vi "Find_Full_Equal_Points-1.vi"(4 "error IN":errorcluster, 5 "[IN] Activate Search???":bool, 7 "[IN] Clusters for Re\nconstructed Tracks":T1) -> (0 "error OUT":errorcluster, 3 "[OUT] Clusters for Re\nconstructed Tracks":T1)   [LabVIEW 2017]
panel:
  out "# of Track":i32
  out "Index in Track":i32
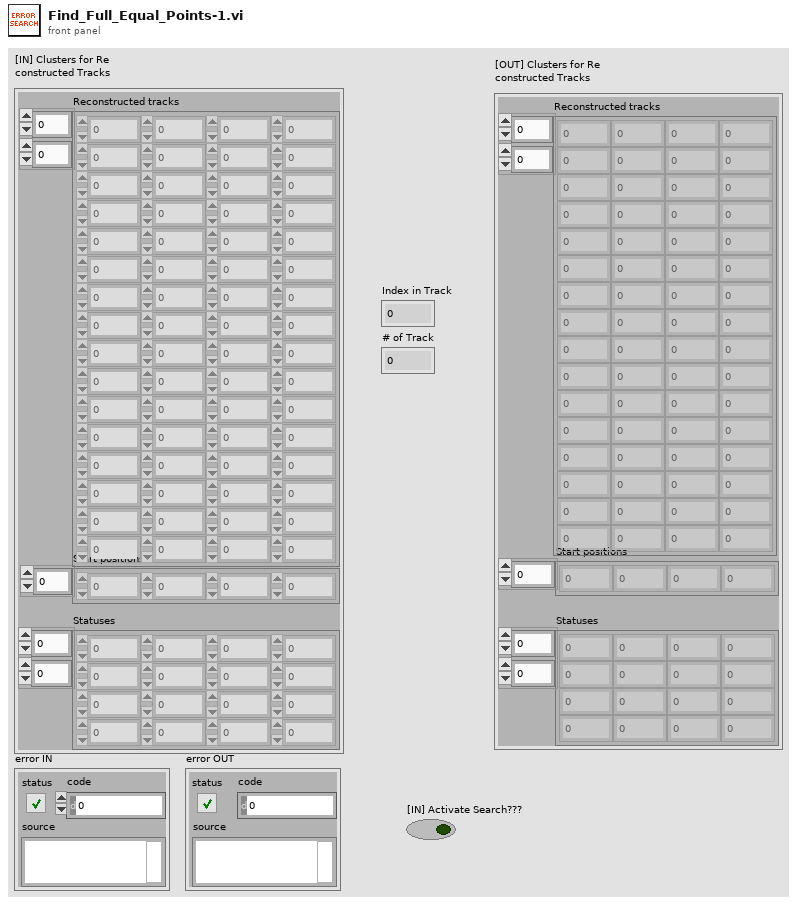
[diagram p1: front panel]
types:
  T1 = cluster{"Reconstructed tracks":dbl[][], "Start positions":i32[], "Statuses":i16[][]}
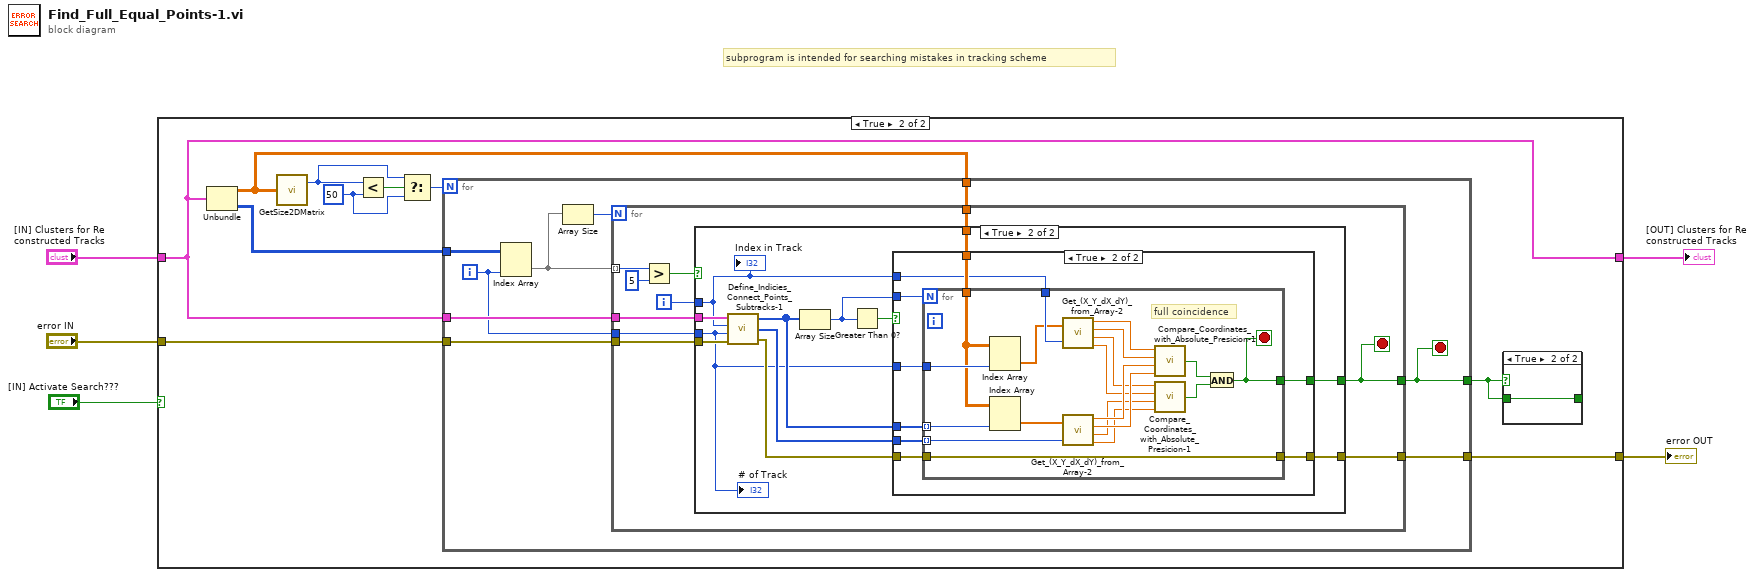
[diagram p0: block diagram]
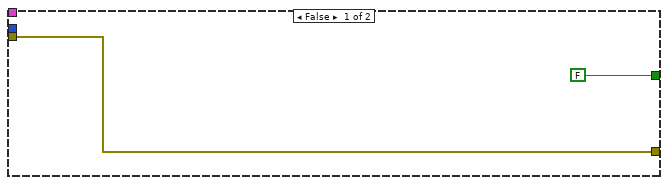
[diagram p4: hidden frame]
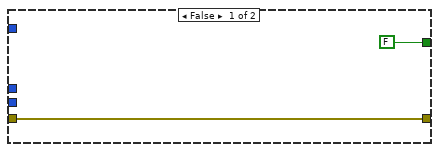
[diagram p5: hidden frame]
diagram:
  # "subprogram is intended for searching mistakes in tracking scheme"
  n1 = case shown="True" "[IN] Activate Search???" {
    tunnel: "[IN] Clusters for Re\nconstructed Tracks" -> [w6 w8]
    tunnel: "error IN" -> [w7 w12]
    tunnel: [w7 w10] -> w2
    tunnel: [w6 w8] -> w1
    frame False {
    }
    frame True {
      w15 = 50 ("y")
      n2 = Unbundle(w8) -> ("Reconstructed tracks"=w11:dbl[][], "Statuses"=w13:i16[][])  [unwired: 1 out]
      n3 = call "GetSize2DMatrix.vi"("Array IN (2D)"=w11) -> ("# Cols"=w16:i32)  [unwired: 1 out]
      n4 = Less?(x=w16, y=w15) -> (x < y?=w17:bool)
      n5 = Select(t=w16, s=w17, f=w15) -> (s? t:f=w14:i32)
      n6 = for {
        N: w14 -> [_]
        tunnel: w13 -> [w28]
        tunnel: w8 -> [w25]
        tunnel: w12 -> [w24]
        tunnel: w11 -> [w22]
        tunnel: [w21] -> w9
        tunnel: [w20] -> w10
        i -> [w23]
        stop <- w21 stop-if-true
        n7 = Index Array(array=w28, index (col)=w23) -> (element=w26:i16[])  [unwired: 1 in]
        n8 = Array Size(array=w26) -> (size(s)=w27:i32)
        n9 = for {
          N: w27 -> [_]
          tunnel: w26 -> [w34] mode=indexing
          tunnel: w25 -> [w36]
          tunnel: w24 -> [w35]
          tunnel: w23 -> [w32]
          tunnel: w22 -> [w31]
          tunnel: [w30] -> w21
          tunnel: [w29] -> w20
          i -> [w33]
          stop <- w30 stop-if-true
          n10 = Greater?(x=w34, y=i16 5) -> (0:w37:bool)
          n11 = case shown="True" w37 {
            tunnel: w36 -> [_ w52]
            tunnel: w35 -> [w39 w51]
            tunnel: w33 -> [_ w43]
            tunnel: w32 -> [_ w44]
            tunnel: w31 -> [_ w45]
            tunnel: [FALSE w42] -> w30
            tunnel: [w39 w41] -> w29
            frame False {
            }
            frame True {
              n12 = call "Define_Indicies_Connect_Points_Subtracks-1.vi"("error IN"=w51, "[IN] Index of track with\n(problem displacement)"=w44, "[IN] Index of problem\ndisplacement inside track"=w43, "[IN] Track group"=w52) -> ("error OUT"=w46:errorcluster, "[OUT] Index of \nconnected dots\ninside the track"=w47:i32[], "[OUT] Index of connected\ntracks with problem dot"=w48:i32[])
              n13 = Array Size(array=w48) -> (size(s)=w50:i32)
              n14 = Greater Than 0?(x=w50) -> (x > 0?=w49:bool)
              n15 = case shown="True" w49 {
                tunnel: w50 -> [_ w63]
                tunnel: w48 -> [_ w62]
                tunnel: w47 -> [_ w61]
                tunnel: w46 -> [w53 w60]
                tunnel: w45 -> [_ w59]
                tunnel: w44 -> [_ w58]
                tunnel: w43 -> [_ w57]
                tunnel: [FALSE w56] -> w42
                tunnel: [w53 w55] -> w41
                frame False {
                }
                frame True {
                  n16 = for {
                    N: w63 -> [_]
                    tunnel: w62 -> [w78] mode=indexing
                    tunnel: w61 -> [w76] mode=indexing
                    tunnel: w60 -> [w65]
                    tunnel: w59 -> [w79]
                    tunnel: w58 -> [w82]
                    tunnel: w57 -> [w81]
                    tunnel: [w64] -> w56
                    tunnel: [w65] -> w55
                    stop <- w64 stop-if-true
                    # "full coincidence"
                    n17 = Index Array(array=w79, index (col)=w82) -> (element=w80:dbl[])  [unwired: 1 in]
                    n18 = Index Array(array=w79, index (col)=w78) -> (element=w77:dbl[])  [unwired: 1 in]
                    n19 = call "Get_(X_Y_dX_dY)_from_Array-2.vi"("(X,Y,dX,dY)"=w80, "Index of Displacement"=w81) -> ("X"=w75:dbl, "Y"=w74:dbl, "dX"=w71:dbl, "dY"=w70:dbl)
                    n20 = call "Get_(X_Y_dX_dY)_from_Array-2.vi"("(X,Y,dX,dY)"=w77, "Index of Displacement"=w76) -> ("X"=w73:dbl, "Y"=w72:dbl, "dX"=w69:dbl, "dY"=w68:dbl)
                    n21 = call "Compare_Coordinates_with_Absolute_Presicion-1.vi"("X 1"=w75, "Y 1"=w74, "X 2"=w73, "Y 2"=w72) -> ("[OUT] Same coordinates?"=w67:bool)  [unwired: 1 in]
                    n22 = call "Compare_Coordinates_with_Absolute_Presicion-1.vi"("X 1"=w71, "Y 1"=w70, "X 2"=w69, "Y 2"=w68) -> ("[OUT] Same coordinates?"=w66:bool)  [unwired: 1 in]
                    n23 = And(x=w67, y=w66) -> (x .and. y?=w64:bool)
                  }
                }
              }
              "Index in Track" <- w43
              "# of Track" <- w44
            }
          }
        }
      }
      n24 = case shown="True" w9 {
        tunnel: w9 -> [w18 w19]
        tunnel: [w18 w19] -> _
        frame False {
        }
        frame True {
        }
      }
    }
  }
  "error OUT" <- w2
  "[OUT] Clusters for Re\nconstructed Tracks" <- w1
